vi "Temperature To Text Color.vi"(8 "Lower Limit":dbl, 9 "Temperature":dbl format="%#_13g", 10 "Upper Limit":dbl, 11 "reference":refnum<vi>) -> ()   [LabVIEW 2019, in "Personalities Tool.lvlib"]
uses:
  Personalities Tool.lvlib
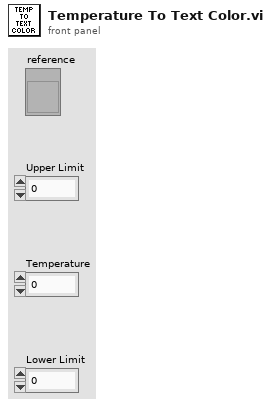
[diagram p1: front panel]
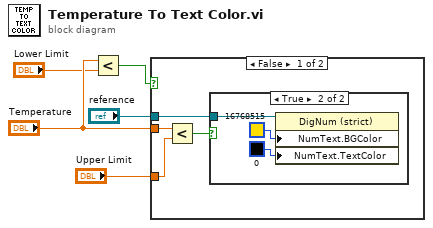
[diagram p0: block diagram]
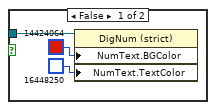
[diagram p2: hidden frame]
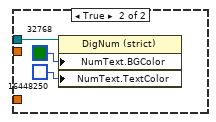
[diagram p3: hidden frame]
diagram:
  n1 = Less?(x="Temperature", y="Lower Limit") -> (x < y?=w5:bool)
  n2 = case shown="False" w5 {
    tunnel: "Temperature" -> [w7 _]
    tunnel: "Upper Limit" -> [w9 _]
    tunnel: "reference" -> [w6 w16]
    frame False {
      n3 = Less?(x=w7, y=w9) -> (x < y?=w8:bool)
      n4 = case shown="True" w8 {
        tunnel: w6 -> [w10 w13]
        frame False {
          n5 = property on="Property Node" class="DigNum (strict)"(reference=w10, "NumText.BGColor"=u32 14424064, "NumText.TextColor"=u32 16448250) -> ()  [unwired: 1 in, 2 out]
        }
        frame True {
          n6 = property on="Property Node" class="DigNum (strict)"(reference=w13, "NumText.BGColor"=u32 16768515, "NumText.TextColor"=u32 0) -> ()  [unwired: 1 in, 2 out]
        }
      }
    }
    frame True {
      n7 = property on="Property Node" class="DigNum (strict)"(reference=w16, "NumText.BGColor"=u32 32768, "NumText.TextColor"=u32 16448250) -> ()  [unwired: 1 in, 2 out]
    }
  }
